vi "HMF2500 Set Frequency.vi"(8 "error in (no error)":errorcluster, 10 "frequency [Hz] (1000)":dbl=1000.0, 11 "VISA in":refnum<visa-resource-name>) -> (0 "error out":errorcluster, 3 "VISA out":refnum<visa-resource-name>)   [LabVIEW 2020, in "AWG.lvlib"]
doc: "Set output frequency."
uses:
  AWG.lvlib
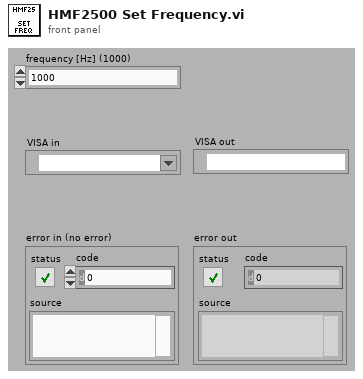
[diagram p1: front panel]
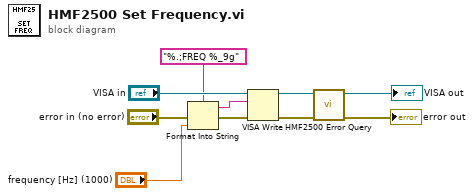
[diagram p0: block diagram]
diagram:
  n1 = Format Into String(format string="%.;FREQ %_9g", error in="error in (no error)", "frequency [Hz] (1000)") -> (resulting string=w8:string, error out=w9:errorcluster)  [unwired: 1 in]
  n2 = VISA Write(VISA resource name="VISA in", write buffer=w8, error in (no error)=w9) -> (VISA resource name out=w4:refnum<visa-resource-name>, error out=w5:errorcluster)  [unwired: 1 out]
  n3 = call "HMF2500 Error Query.vi"("error in (no error)"=w5, "VISA resource name"=w4) -> ("error out"=→"error out":errorcluster, "VISA resource name out"=→"VISA out":refnum<visa-resource-name>)  [unwired: 6 in, 2 out]
